vi "Acquire Data.vi"(8 "error in (no error)":errorcluster, 11 "Camera in":refnum<class "Camera.lvclass">) -> (0 "error out":errorcluster, 3 "Camera out":refnum<class "Camera.lvclass">)   [LabVIEW 2020, in "Camera.lvclass"]
uses:
  Camera.lvclass
  Sensor.lvclass
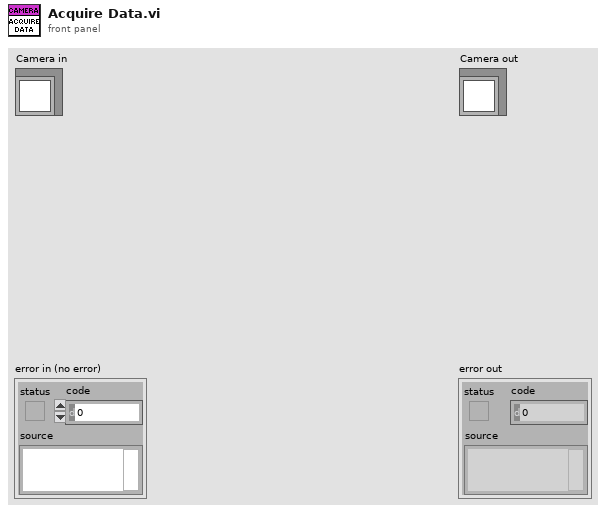
[diagram p1: front panel]
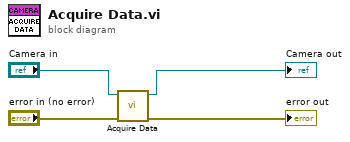
[diagram p0: block diagram]
diagram:
  n1 = call-parent "Acquire Data.vi"("error in (no error)"="error in (no error)", "Sensor in"="Camera in") -> ("error out"=→"error out":errorcluster, "Sensor out"=→"Camera out":refnum<class "Camera.lvclass">)  [unwired: 8 in]
